vi "ITX Decimation.vi"(0 "file (use dialog)":path=path "P:/sample/GaAs/GaAs quantum dots/2008/PL Map/A1 735/060731ASBA_A1_6.0.itx") -> (4 "wave names":string[](array[string]), 5 "Notes":string)   [LabVIEW 2013]
uses:
  <vilib>/Analysis/2dsp.llb/Decimate (single shot, DBL).vi
  <vilib>/Analysis/NI_AALPro.lvlib
panel:
  in  "Decimating Factor":i32=400
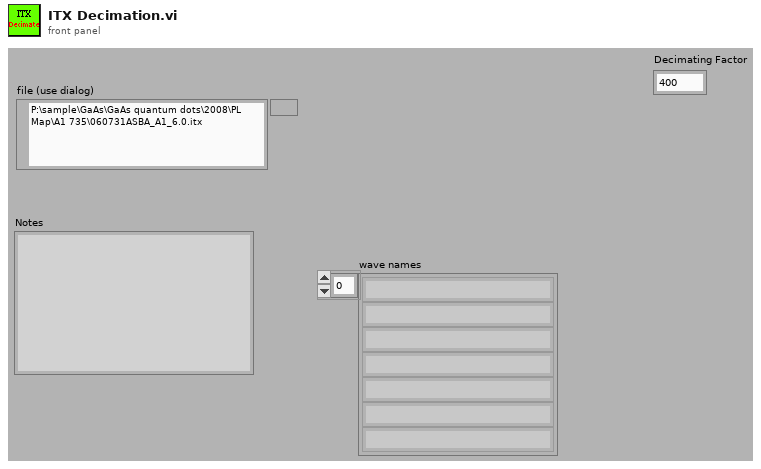
[diagram p1: front panel]
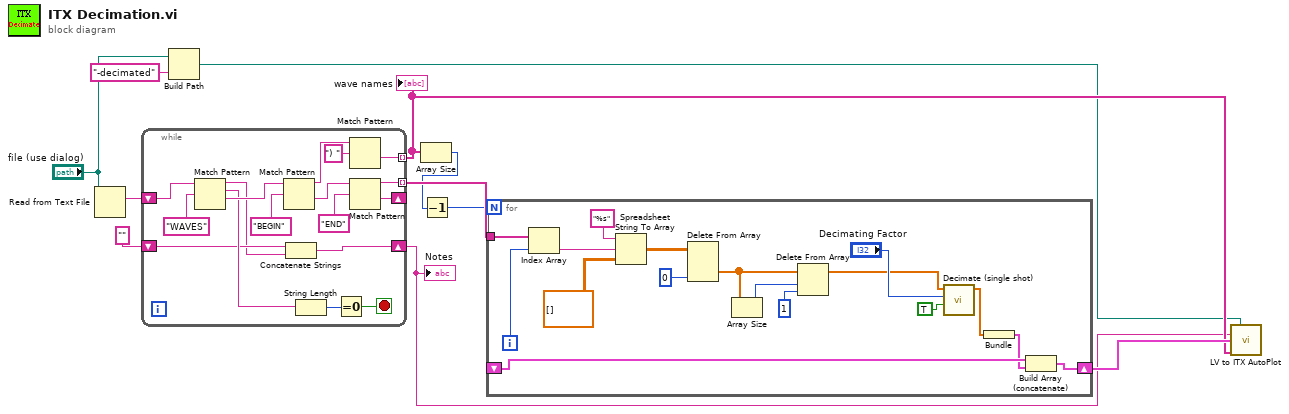
[diagram p0: block diagram]
diagram:
  n1 = Read from Text File(file (use dialog)="file (use dialog)") -> (text=w11:string)  [unwired: 2 in, 4 out]
  n2 = while {
    tunnel: [w12] -> w9 mode=indexing
    shift-right: [w26] -> _
    shift-left: w11 -> [w14]
    tunnel: [w22] -> w5 mode=indexing
    shift-right: [w17] -> w4
    shift-left: "" ("regular expression") -> [w16]
    stop <- w23 stop-if-true
    n3 = Match Pattern(string=w14, regular expression="WAVES") -> (before substring=w15:string, match substring=w25:string, after substring=w28:string)  [unwired: 2 out]
    n4 = Match Pattern(string=w28, regular expression="BEGIN" ("regular expression 2")) -> (before substring=w13:string, after substring=w27:string)  [unwired: 3 out]
    n5 = Concatenate Strings(w16, w15) -> (w17:string)
    n6 = String Length(string=w25) -> (length=w24:i32)
    n7 = Equal To 0?(x=w24) -> (x = 0?=w23:bool)
    n8 = Match Pattern(string=w13, regular expression=") ") -> (after substring=w22:string)  [unwired: 4 out]
    n9 = Match Pattern(string=w27, regular expression="END" ("regular expression 3")) -> (before substring=w12:string, after substring=w26:string)  [unwired: 3 out]
  }
  "wave names" <- w5
  "Notes" <- w4
  n10 = Build Path(base path="file (use dialog)", name or relative path="-decimated") -> (appended path=w1:path)
  n11 = Array Size(array=w5) -> (size(s)=w8:i32)
  n12 = Decrement(x=w8) -> (x-1=w7:i32)
  n13 = for {
    N: w7 -> [_]
    tunnel: w9 -> [w40]
    shift-right: [w32] -> w6
    shift-left: _ -> [w31]
    i -> [w36]
    n14 = Index Array(array=w40, index=w36) -> (element=w39:string)
    n15 = Spreadsheet String To Array(format string="%s", spreadsheet string=w39, array type (2D Dbl)=dbl[][] []) -> (array=w44:dbl[][])  [unwired: 1 out]
    n16 = Delete From Array(array=w44, index (col)=0 ("disabled index (col)")) -> (deleted portion=w43:dbl[])  [unwired: 2 in, 1 out]
    n17 = Array Size(array=w43) -> (size(s)=w42:i32)
    n18 = Delete From Array(array=w43, length=w42, index=1) -> (array with subset deleted=w33:dbl[])  [unwired: 1 out]
    n19 = call-poly <vilib>:"Decimate (single shot).vi"("averaging"=TRUE, "decimating factor"="Decimating Factor", "X"=w33) -> ("Decimated Array"=w29:dbl[])  [unwired: 7 in, 1 out]
    n20 = Bundle("Decimated Array"=w29) -> (w30:cluster{"Decimated Array":dbl[]})  [unwired: 1 in]
    n21 = Build Array (concatenate)(w31, w30) -> (w32:cluster{"Decimated Array":dbl[]}[])
  }
  n22 = call <userlib>:"LV to ITX AutoPlot.vi"("path"=w1, "Notes"=w4, "Data"=w6, "wavenames (.Vx, etc)"=w5) -> ()  [unwired: 11 in, 1 out]
